vi "Read KickAngle.vi"(8 "error in (no error)":errorcluster, 11 "Parameters in":refnum<class "Parameters.lvclass">) -> (0 "error out":errorcluster, 2 "KickAngle":dbl=0.09, 3 "Parameters out":refnum<class "Parameters.lvclass">)   [LabVIEW 2023, in "Parameters.lvclass"]
uses:
  Parameters.lvclass
  Parameters.lvclass/Parameters.ctl
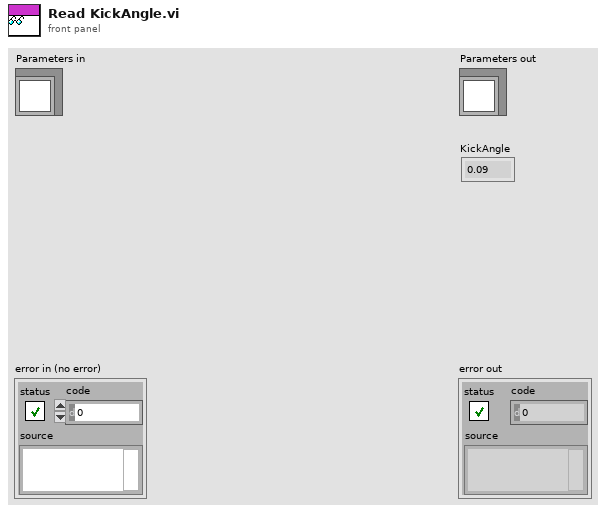
[diagram p1: front panel]
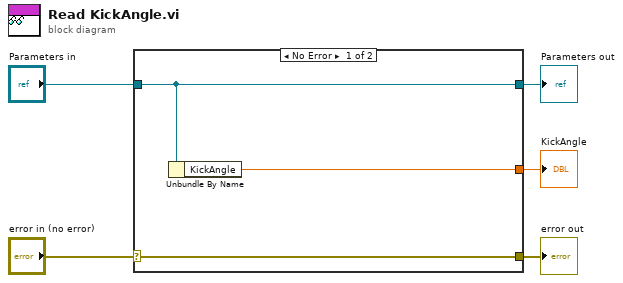
[diagram p0: block diagram]
diagram:
  n1 = case shown="No Error" "error in (no error)" {
    selector: "error in (no error)" -> [w8 w9]
    tunnel: [w8 w9] -> w4
    tunnel: [w7 w10] -> w2
    tunnel: "Parameters in" -> [w7 w10]
    tunnel: [w6 _] -> w1
    frame No Error {
      n2 = Unbundle By Name(w7) -> ("KickAngle"=w6:dbl)
    }
    frame Error {
    }
  }
  "error out" <- w4
  "Parameters out" <- w2
  "KickAngle" <- w1
